vi "SetInitialPlayerPositions_Random.vi"(8 "error in (no error)":errorcluster, 11 "Board in":refnum<class "Board.lvclass">) -> (0 "error out":errorcluster, 3 "Board out":refnum<class "Board.lvclass">)   [LabVIEW 2015, in "TronviewGame.lvlib" / "GameBuilder.lvclass"]
uses:
  GameBuilder.lvclass
  Board/Board.lvclass
  Board/Position.ctl
  Board/Board.lvclass/Board.ctl
  Board/GetSize.vi
  Board/GetBoardCenter.vi
  <vilib>/gmath/statdist.llb/Random Permutation.vi
  <vilib>/gmath/NI_Gmath.lvlib
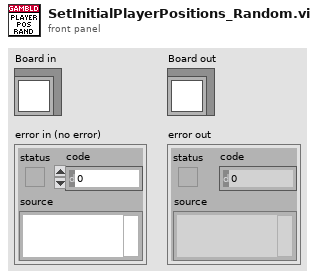
[diagram p1: front panel]
types:
  T1 = typedef "TronviewGame.lvlib/Board.lvclass/Position.ctl" = cluster{"Column":i32, "Row":i32}
  T2 = typedef "TronviewGame.lvlib/Board.lvclass/BoardSize.ctl" = cluster{"Columns":u16, "Rows":u16}
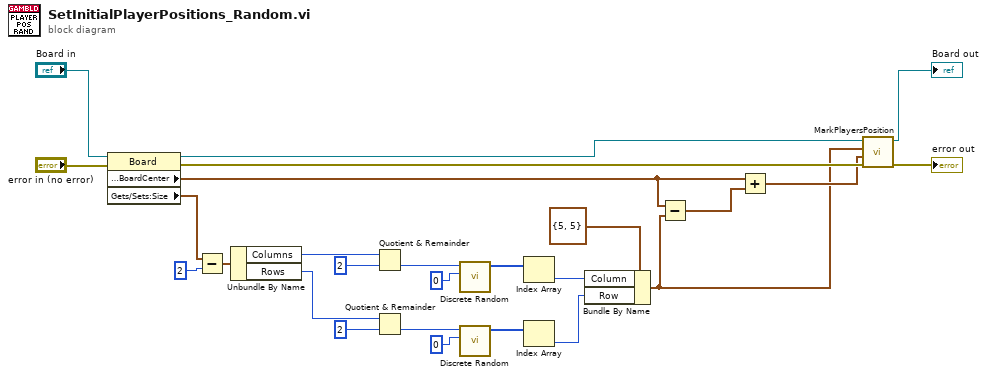
[diagram p0: block diagram]
diagram:
  n1 = property class="Board"(reference="Board in", error in="error in (no error)") -> (reference out=w20:refnum<class "Board.lvclass">, error out=w22:errorcluster, "Gets/Sets:BoardCenter"=w25:T1, "Gets/Sets:Size"=w2:T2)
  n2 = Subtract(x=w2, y=u16 2) -> (x-y=w3:T2)
  n3 = Unbundle By Name(w3) -> ("Columns"=w15:u16, "Rows"=w7:u16)
  n4 = Quotient & Remainder(x=w15, y=u16 2) -> (floor(x/y)=w14:u16)  [unwired: 1 out]
  n5 = Quotient & Remainder(x=w7, y=u16 2) -> (floor(x/y)=w6:u16)  [unwired: 1 out]
  n6 = call-poly <vilib>:"Discrete Random.vi"("start"=0, "N"=w14) -> ("random permutation"=w12:i32[])  [unwired: 8 in, 1 out]
  n7 = call-poly <vilib>:"Discrete Random.vi"("start"=0, "N"=w6) -> ("random permutation"=w5:i32[])  [unwired: 8 in, 1 out]
  n8 = Index Array(array=w12) -> (element=w10:i32)  [unwired: 1 in]
  n9 = Index Array(array=w5) -> (element=w4:i32)  [unwired: 1 in]
  n10 = Bundle By Name(cluster=T1 {"Column"=5, "Row"=5} ("Position"), "Column"=w10, "Row"=w4) -> (w11:T1)
  n11 = Subtract(x=w25, y=w11) -> (x-y=w24:T1)
  n12 = Add(x=w25, y=w24) -> (x+y=w19:T1)
  n13 = call "MarkPlayersPosition.vi"("error in (no error)"=w22, "Player2NewPosition"=w19, "Player1NewPosition"=w11, "Board in"=w20) -> ("error out"=→"error out":errorcluster, "Board out"=→"Board out":refnum<class "Board.lvclass">)  [unwired: 4 in, 2 out]
